vi "mono_sensor_init.vi"(8 "error in (no error)":errorcluster, 11 "Cluster in":T1) -> (3 "Cluster out":T2)   [LabVIEW 2018]
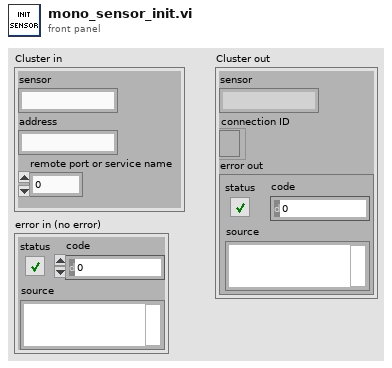
[diagram p1: front panel]
types:
  T1 = cluster{"sensor":string, "address":string, "remote port or service name":u16}
  T2 = cluster{"sensor":string, "connection ID":refnum<k5>, "error out":errorcluster}
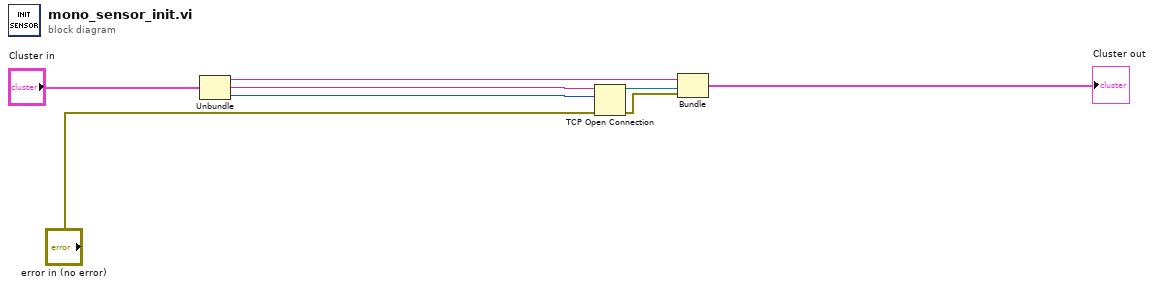
[diagram p0: block diagram]
diagram:
  n1 = Unbundle("Cluster in") -> ("sensor"=w6:string, "address"=w2:string, "remote port or service name"=w3:u16)
  n2 = TCP Open Connection(address=w2, remote port or service name=w3, error in (no error)="error in (no error)") -> (connection ID=w7:refnum<k5>, error out=w8:errorcluster)  [unwired: 2 in]
  n3 = Bundle("sensor"=w6, "connection ID"=w7, "error out"=w8) -> (→"Cluster out":T2)  [unwired: 1 in]
